vi "list_stored_positions.vi"(8 "error in (no error)":errorcluster, 11 "StageDL090409Scaffold in":refnum<class "StageDL090409Scaffold.lvclass">) -> (0 "error out":errorcluster, 3 "StageDL090409Scaffold out":refnum<class "StageDL090409Scaffold.lvclass">)   [LabVIEW 2010, in "StageDL090409Scaffold.lvclass"]
uses:
  StageDL090409Scaffold.lvclass
  StageDL090409Scaffold.lvclass/StageDL090409Scaffold.ctl
  common/classes/SpaceVector/SpaceVector/SpaceVector.lvclass
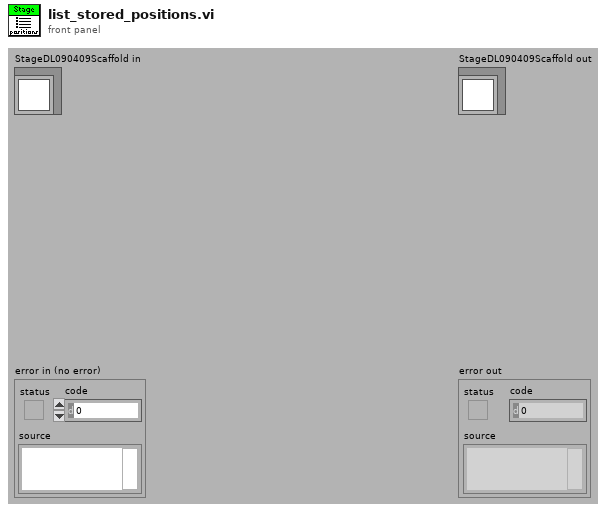
[diagram p1: front panel]
types:
  T1 = typedef "StageDL090409Scaffold.lvclass/stored_data_cluster.ctl" = cluster{"stored position":refnum<class "SpaceVector.lvclass">, "description":string, "position image":refnum<class "Image.lvclass">}
  T2 = typedef "space_vector_array.ctl" = dbl[unit][]
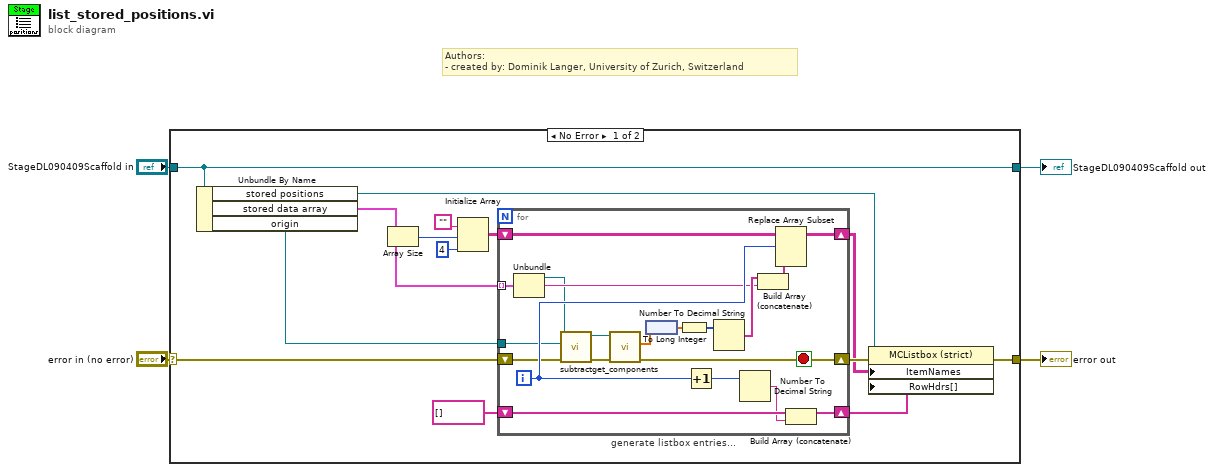
[diagram p0: block diagram]
diagram:
  # "Authors: \n- created by: Dominik Langer, University of Zurich, Switzerland"
  n1 = case shown="No Error" "error in (no error)" {
    selector: "error in (no error)" -> [w10 w40]
    tunnel: [w9 w40] -> w3
    tunnel: [w8 w39] -> w1
    tunnel: "StageDL090409Scaffold in" -> [w8 w39]
    frame No Error {
      n2 = Unbundle By Name(w8) -> ("stored positions"=w6:refnum<vi>, "stored data array"=w7:T1[], "origin"=w5:refnum<class "SpaceVector.lvclass">)
      n3 = Array Size(array=w7) -> (size(s)=w12:i32)
      n4 = Initialize Array("", w12, 4 ("dimension size")) -> (w16:string[][])
      n5 = for "generate listbox entries..." {
        tunnel: w7 -> [w38] mode=indexing
        shift-right: [w30] -> w14
        shift-left: w16 -> [w37]
        shift-right: [w36] -> w13
        shift-left: string[] [] -> [w35]
        shift-right: [w31] -> w15
        shift-left: w10 -> [w24]
        tunnel: w5 -> [w22]
        i -> [w34]
        stop <- w31 stop-if-true
        n6 = Unbundle(w38) -> ("stored position"=w26:refnum<class "SpaceVector.lvclass">, "description"=w28:string)  [unwired: 1 out]
        n7 = call "subtract.vi"("error in (no error)"=w24, "subtrahend"=w22, "SpaceVector in"=w26) -> ("error out"=w23:errorcluster, "SpaceVector out"=w25:refnum<class "SpaceVector.lvclass">)  [unwired: 7 in]
        n8 = call "get_components.vi"("error in (no error)"=w23, "SpaceVector in"=w25) -> ("error out"=w31:errorcluster, "x/y/z"=w21:T2)  [unwired: 4 in, 4 out]
        n9 = node(w21) -> (w20:dbl[])
        n10 = To Long Integer(number=w20) -> (32bit integer=w19:i32[])
        n11 = Increment(x=w34) -> (x+1=w33:i32)
        n12 = Number To Decimal String(number=w19) -> (decimal integer string=w29:string[])  [unwired: 1 in]
        n13 = Number To Decimal String(number=w33) -> (decimal integer string=w32:string)  [unwired: 1 in]
        n14 = Build Array (concatenate)(w29, w28) -> (w27:string[])
        n15 = Replace Array Subset(array=w37, new element=w27, index (row)=w34) -> (w30:string[][])  [unwired: 1 in]
        n16 = Build Array (concatenate)(w35, w32) -> (w36:string[])
      }
      n17 = property on="Property Node" class="MCListbox (strict)"(reference=w6, error in=w15, "ItemNames"=w14, "RowHdrs[]"=w13) -> (error out=w9:errorcluster)  [unwired: 1 out]
    }
    frame Error {
    }
  }
  "error out" <- w3
  "StageDL090409Scaffold out" <- w1
